vi "Create_Object.vi"(8 "error in (no error)":errorcluster, 9 "Block Diagram in":T1, 10 "owner refnum":variant, 11 "MultiDiagramStructure in":refnum<class "MultiDiagramStructure.lvclass">) -> (0 "error out":errorcluster, 1 "Block Diagram Out":T1, 3 "MultiDiagramStructure out":refnum<class "MultiDiagramStructure.lvclass">)   [LabVIEW 2025, in "MultiDiagramStructure.lvclass"]
uses:
  MultiDiagramStructure.lvclass
  C:/Users/mrjak/Documents/GitHub/LVGPT/LabVIEW/VIs/Classes/Node/Node.lvclass
  Controls/bd.ctl
  Node.lvclass
  Controls/wire.ctl
  Controls/Terminal.ctl
  Structure.lvclass
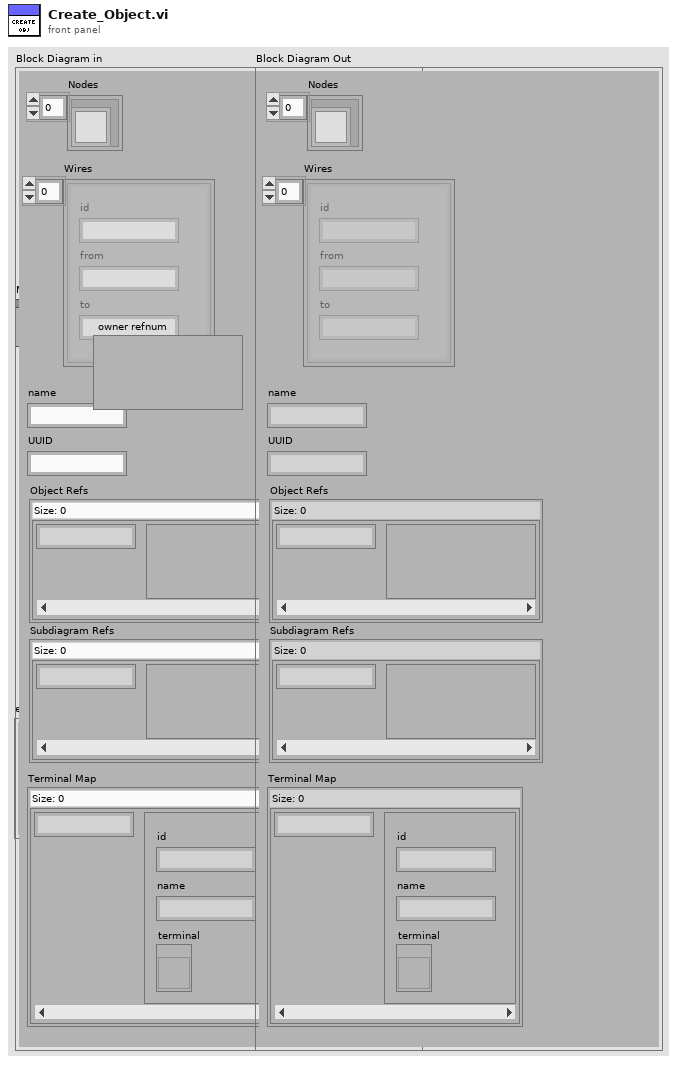
[diagram p1: front panel]
types:
  T1 = typedef "bd.ctl" = cluster{"Nodes":refnum<class "Node.lvclass">[], "Wires":T2[], "name":string, "UUID":string, "Object Refs":map{string, variant}, "Subdiagram Refs":map{string, variant}, "Terminal Map":map{string, T3}}
  T2 = typedef "wire.ctl" = cluster{"id":string, "from":string, "to":string}
  T3 = typedef "Terminal.ctl" = cluster{"id":string, "name":string, "terminal":refnum<vi>}
  T4 = typedef "Subdiagram.ctl" = cluster{"diagram":refnum<vi>, "selector":string, "uuid":string}
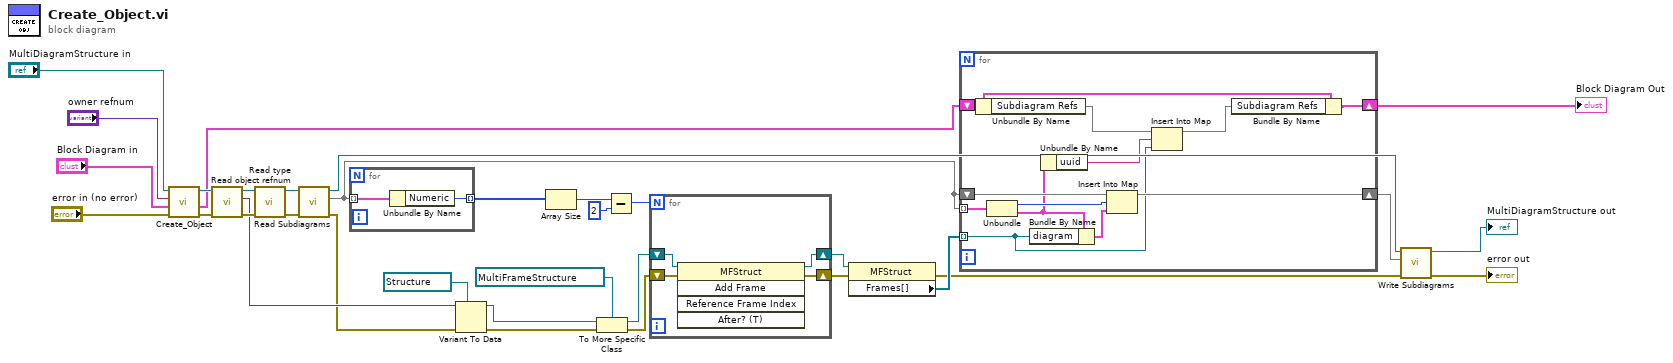
[diagram p0: block diagram]
diagram:
  n1 = call-parent "Create_Object.vi"("error in (no error)"="error in (no error)", "Block Diagram in"="Block Diagram in", "owner refnum"="owner refnum", "Structure in"="MultiDiagramStructure in") -> ("error out"=w30:errorcluster, "Block Diagram Out"=w2:T1, "Structure out"=w29:refnum<class "MultiDiagramStructure.lvclass">)  [unwired: 5 in]
  n2 = call-dynamic "Read object refnum.vi"("error in (no error)"=w30, "Node in"=w29) -> ("error out"=w27:errorcluster, "object refnum"=w10:variant, "Node out"=w28:refnum<class "MultiDiagramStructure.lvclass">)  [unwired: 7 in]
  n3 = call "Read type.vi"("error in (no error)"=w27, "Node in"=w28) -> ("error out"=w11:errorcluster, "Node out"=w22:refnum<class "MultiDiagramStructure.lvclass">)  [unwired: 7 in, 1 out]
  n4 = call-dynamic "Read Subdiagrams.vi"("error in (no error)"=w11, "Structure in"=w22) -> ("error out"=w9:errorcluster, "Subdiagrams"=w17:map{u64, T4}, "Structure out"=w13:refnum<class "MultiDiagramStructure.lvclass">)  [unwired: 7 in]
  n5 = for {
    tunnel: w17 -> [w35] mode=indexing
    tunnel: [w34] -> w18 mode=indexing
    n6 = Unbundle By Name(w35) -> ("Numeric"=w34:u64)
  }
  n7 = Variant To Data(error in=w9, type=refnum<vi> refnum ("vi object class"), Variant=w10) -> (data=w5:refnum<vi>, error out=w8:errorcluster)
  n8 = Array Size(array=w18) -> (size(s)=w19:i32)
  n9 = To More Specific Class(target class=refnum<vi> refnum ("vi object class"), reference=w5, error in=w8) -> (specific class reference=w25:refnum<vi>, error out=w15:errorcluster)
  n10 = Subtract(x=w19, y=2) -> (x-y=w21:i32)
  n11 = for {
    N: w21 -> [_]
    shift-right: [w38] -> w16
    shift-left: w25 -> [w39]
    shift-right: [w36] -> w14
    shift-left: w15 -> [w37]
    n12 = invoke class="MFStruct" method="Add Frame"(reference=w39, error in=w37) -> (reference out=w38:refnum<vi>, error out=w36:errorcluster)  [unwired: 3 in, 3 out]
  }
  n13 = property class="MFStruct"(reference=w16, error in=w14) -> (error out=w12:errorcluster, "Frames[]"=w24:refnum<vi>[])  [unwired: 1 out]
  n14 = for {
    tunnel: w24 -> [w40] mode=indexing
    tunnel: w17 -> [w51] mode=indexing
    shift-right: [w47] -> w23
    shift-left: w17 -> [w50]
    shift-right: [w45] -> w1
    shift-left: w2 -> [w46]
    n15 = Unbundle By Name(w46) -> ("Subdiagram Refs"=w44:map{string, variant})
    n16 = Unbundle(w51) -> ("Numeric"=w48:u64, "Subdiagram"=w42:T4)
    n17 = Bundle By Name(cluster=w42, "diagram"=w40) -> (w49:T4)
    n18 = Unbundle By Name(w42) -> ("uuid"=w41:string)
    n19 = Insert Into Map(map in=w50, key=w48, value=w49) -> (map out=w47:map{u64, T4})  [unwired: 2 out]
    n20 = Insert Into Map(map in=w44, key=w41, value=w40) -> (map out=w43:map{string, variant})  [unwired: 2 out]
    n21 = Bundle By Name(cluster=w46, "Subdiagram Refs"=w43) -> (w45:T1)
  }
  "Block Diagram Out" <- w1
  n22 = call-dynamic "Write Subdiagrams.vi"("error in (no error)"=w12, "Subdiagrams"=w23, "Structure in"=w13) -> ("error out"=→"error out":errorcluster, "Structure out"=→"MultiDiagramStructure out":refnum<class "MultiDiagramStructure.lvclass">)  [unwired: 7 in]
